vi "Runner_Enter.vi"(8 "error in":errorcluster) -> (0 "error out":errorcluster, 3 "Runner's Data OUT":T1)   [LabVIEW 2025]
uses:
  Controls/Runner_Data_Structure.ctl
panel:
  out "Boolean":bool=TRUE
  in  "OK":bool
  in  "Runner's Data IN":T1
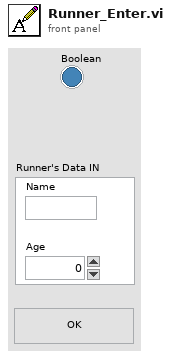
[diagram p1: front panel]
types:
  T1 = typedef "Runner_Data_Structure.ctl" = cluster{"Name":string, "Age":i32}
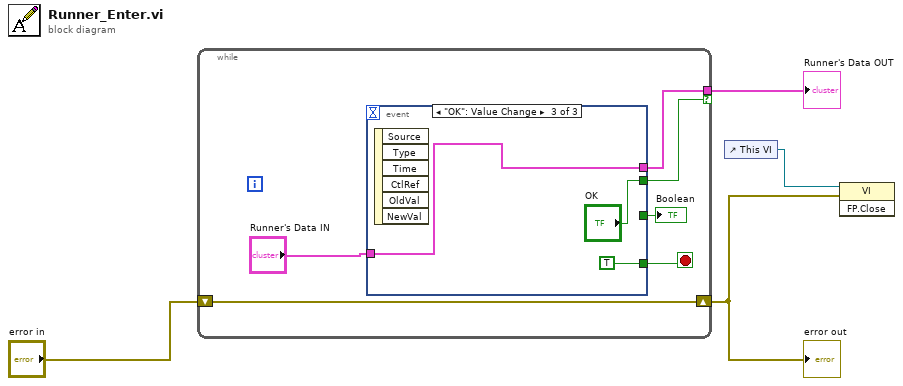
[diagram p0: block diagram]
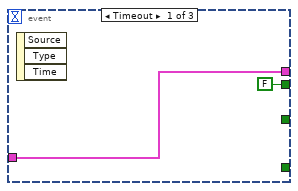
[diagram p2: hidden frame]
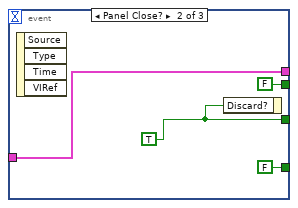
[diagram p3: hidden frame]
diagram:
  n1 = while {
    tunnel: [w9] -> w4 if=w8
    shift-right: [w5] -> w1
    shift-left: "error in" -> [w5]
    stop <- w7 stop-if-true
    n2 = event shown="[2] \"OK\": Value Change" {
      selector: _ -> [_ _ _]
      dyn-events: _ -> [_ _ _]
      timeout: _ -> [_ _ _]
      tunnel: [w12 w14 w19] -> w9
      tunnel: "Runner's Data IN" -> [w12 w14 w19]
      tunnel: [FALSE ("OK") FALSE ("OK") "OK"] -> w8
      tunnel: [_ FALSE TRUE] -> w7
      tunnel: [_ w13 _] -> w6
      event Timeout {
        n3 = event-data() -> ()  [unwired: 1 in, 3 out]
      }
      event Panel Close? {
        w13 = TRUE
        n4 = event-data() -> ()  [unwired: 1 in, 4 out]
        n5 = event-data("Discard?"=w13) -> ()  [unwired: 1 in, 1 out]
      }
      event "OK": Value Change {
        n6 = event-data() -> ()  [unwired: 1 in, 6 out]
      }
    }
    "Boolean" <- w6
  }
  "error out" <- w1
  "Runner's Data OUT" <- w4
  n7 = control-ref of="This VI"() -> (w3:refnum<vi>)
  n8 = invoke class="VI" method="FP.Close"(reference=w3, error in=w1) -> ()  [unwired: 1 in, 3 out]
